vi "SSKIMaxMinAvg(X,N).vi"(10 "X":dbl, 11 "INT_ N":i32) -> (1 "min":dbl, 2 "max":dbl, 3 "AVG(X,N)":dbl, 4 "ix_max":dbl, 6 "ix_min":dbl)   [LabVIEW 2021]
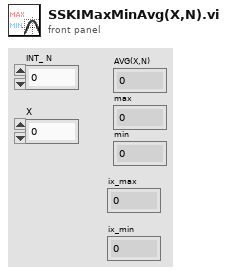
[diagram p1: front panel]
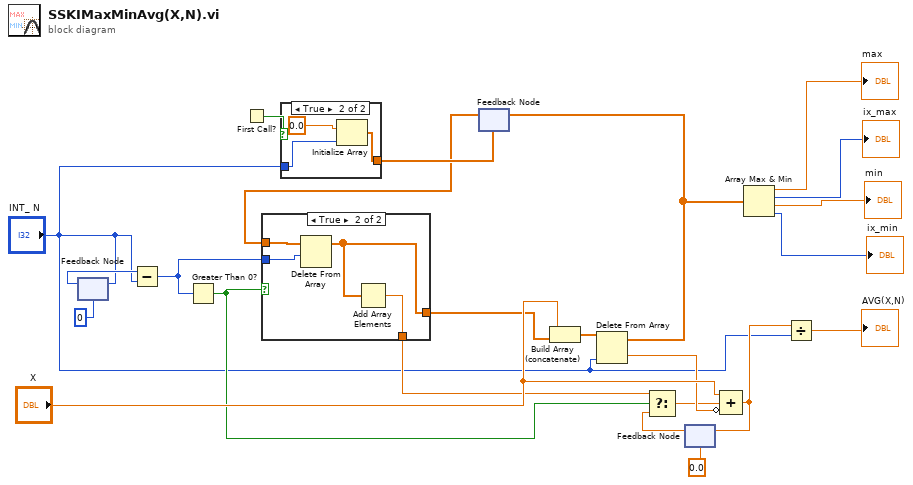
[diagram p0: block diagram]
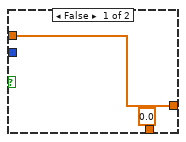
[diagram p2: hidden frame]
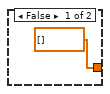
[diagram p3: hidden frame]
diagram:
  n1 = feedback #1(0 ("INT_ N")) -> (w12:i32)
  n2 = feedback-in #1("INT_ N") -> ()
  n3 = Subtract(x=w12, y="INT_ N") -> (x-y=w9:i32)
  n4 = Greater Than 0?(x=w9) -> (x > 0?=w4:bool)
  n5 = First Call?() -> (First Call?: T/F=w23:bool)
  n6 = case shown="True" w23 {
    tunnel: [dbl[] [] w26] -> w22
    tunnel: "INT_ N" -> [_ w25]
    frame False {
    }
    frame True {
      n7 = Initialize Array(0.0 ("element"), w25) -> (w26:dbl[])
    }
  }
  n8 = feedback #2(w22) -> (w10:dbl[])
  n9 = case shown="True" w4 {
    tunnel: [w29 w31] -> w11
    tunnel: w10 -> [w29 w33]
    tunnel: w9 -> [_ w32]
    tunnel: [0.0 ("element") w30] -> w3
    frame False {
    }
    frame True {
      n10 = Delete From Array(array=w33, length=w32) -> (array with subset deleted=w31:dbl[])  [unwired: 1 in, 1 out]
      n11 = Add Array Elements(numeric array=w31) -> (sum=w30:dbl)
    }
  }
  n12 = Build Array (concatenate)("X", w11) -> (w14:dbl[])
  n13 = Delete From Array(array=w14, index="INT_ N") -> (deleted portion=w8:dbl, array with subset deleted=w15:dbl[])  [unwired: 1 in]
  n14 = feedback-in #2(w15) -> ()
  n15 = feedback #3(0.0) -> (w2:dbl)
  n16 = Select(t=w3, s=w4, f=w2) -> (s? t:f=w5:dbl)
  n17 = Compound Arithmetic op=ADD("X", w5, invert w8) -> (w20:dbl)
  n18 = feedback-in #3(w20) -> ()
  n19 = Array Max & Min(array=w15) -> (max value=→"max":dbl, max index (indices)=→"ix_max":i32, min value=→"min":dbl, min index (indices)=→"ix_min":i32)
  n20 = Divide(x=w20, y="INT_ N") -> (x/y=→"AVG(X,N)":dbl)
